vi "Save Best Fit Parameters.vi"(8 "Current File Num":i32, 9 "Best Fit Parameters":dbl[](array[numeric]), 10 "Fitting Results Save Path":string[](array[string]), 11 "Fitting Type":u16(ring)) -> ()   [LabVIEW 2013]
uses:
  <vilib>/Utility/file.llb/Read From Spreadsheet File (DBL).vi
  <vilib>/Utility/file.llb/Write To Spreadsheet File (DBL).vi
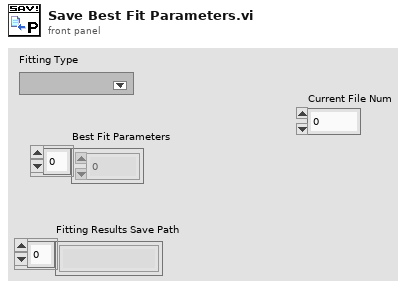
[diagram p1: front panel]
types:
  T1 = enum16{"open", "replace", "create", "open or create", "replace or create", "replace or create with confirmation"}
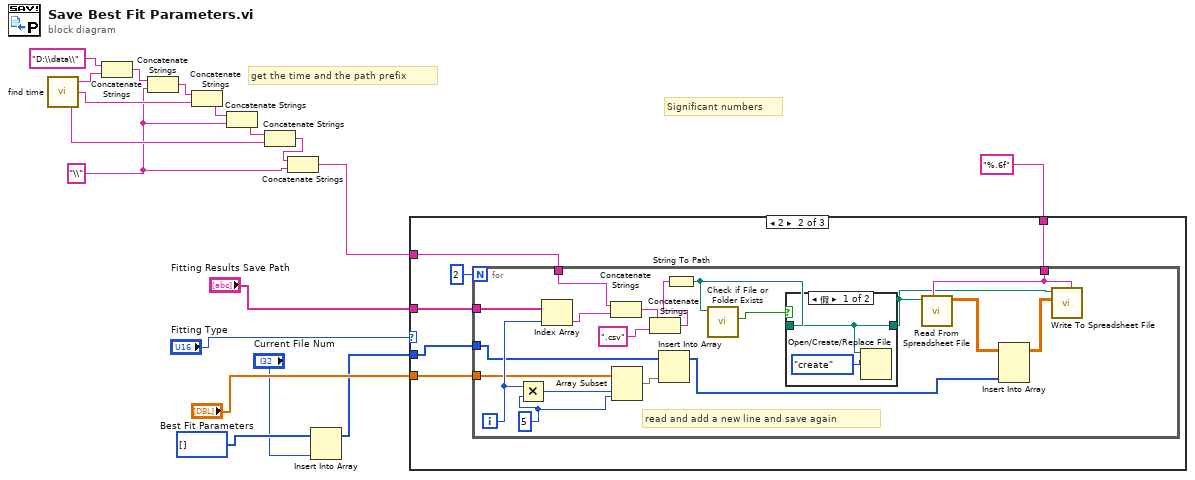
[diagram p0: block diagram]
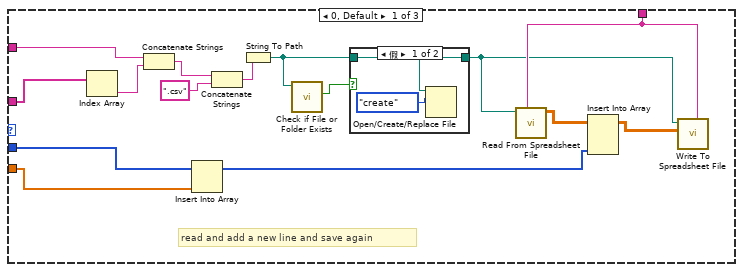
[diagram p2: hidden frame]
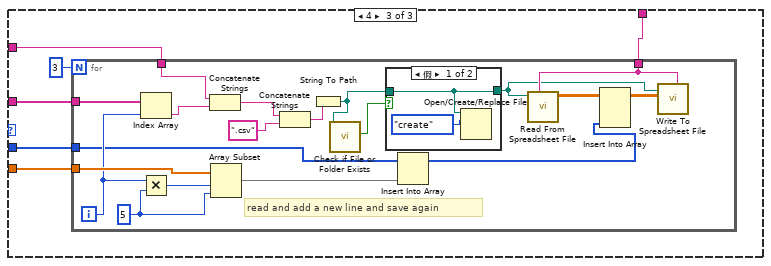
[diagram p5: hidden frame]
diagram:
  w2 = "\\" ("字符串")
  # "get the time and the path prefix"
  # "Significant numbers"
  n1 = call "find time.vi"() -> ("day"=w4:string, "month"=w7:string, "year"=w10:string)  [unwired: 3 in]
  n2 = Concatenate Strings("D:\\data\\", w10) -> (w9:string)
  n3 = Concatenate Strings(w9, w2) -> (w8:string)
  n4 = Concatenate Strings(w8, w7) -> (w6:string)
  n5 = Concatenate Strings(w6, w2) -> (w5:string)
  n6 = Concatenate Strings(w5, w4) -> (w3:string)
  n7 = Concatenate Strings(w3, w2) -> (w1:string)
  n8 = Insert Into Array(array=i32[] [], new element="Current File Num") -> (w13:i32[])  [unwired: 1 in]
  n9 = case shown="2" "Fitting Type" {
    tunnel: "Best Fit Parameters" -> [w28 w41 w69]
    tunnel: "Fitting Results Save Path" -> [w31 w40 w68]
    tunnel: w13 -> [w29 w39 w67]
    tunnel: "%.6f" ("format (%.3f)") -> [w26 w38 w66]
    tunnel: w1 -> [w25 w37 w65]
    frame 0, Default {
      # "read and add a new line and save again"
      n10 = Index Array(array=w31) -> (element=w30:string)  [unwired: 1 in]
      n11 = Concatenate Strings(w25, w30) -> (w23:string)
      n12 = Insert Into Array(array=w29, new element=w28) -> (w27:i32[])  [unwired: 1 in]
      n13 = Concatenate Strings(w23, ".csv" ("字符串")) -> (w22:string)
      n14 = String To Path(string=w22) -> (path=w21:path)
      n15 = call <vilib>:"Check if File or Folder Exists.vi"("path"=w21) -> ("file or folder exists?"=w19:bool)  [unwired: 8 in, 2 out]
      n16 = case shown="假" w19 {
        tunnel: w21 -> [w34 w36]
        tunnel: [w34 w36] -> w20
        frame False {
          n17 = Open/Create/Replace File(file path (use dialog)=w34, operation (0:open)=T1."create" ("操作(0:open)")) -> ()  [unwired: 4 in, 3 out]
        }
        frame True {
        }
      }
      n18 = call-poly <vilib>:"Read From Spreadsheet File.vi"("format (%.3f)"=w26, "file path (dialog if empty)"=w20) -> ("all rows"=w33:dbl[][])  [unwired: 5 in, 4 out]
      n19 = Insert Into Array(array=w33, new element=w27) -> (w32:dbl[][])  [unwired: 2 in]
      n20 = call-poly <vilib>:"Write To Spreadsheet File.vi"("format (%.3f)"=w26, "2D data"=w32, "file path (dialog if empty)"=w20) -> ()  [unwired: 5 in, 1 out]
    }
    frame 2 {
      n21 = for {
        N: 2 -> [_]
        tunnel: w41 -> [w53]
        tunnel: w40 -> [w59]
        tunnel: w39 -> [w54]
        tunnel: w38 -> [w50]
        tunnel: w37 -> [w49]
        i -> [w58]
        w60 = 5 ("x")
        # "read and add a new line and save again"
        n22 = Multiply(x=w58, y=w60) -> (x*y=w61:i32)
        n23 = Index Array(array=w59, index=w58) -> (element=w57:string)
        n24 = Concatenate Strings(w49, w57) -> (w48:string)
        n25 = Array Subset(array=w53, index=w61, length=w60) -> (w52:dbl[])
        n26 = Concatenate Strings(w48, ".csv" ("字符串")) -> (w46:string)
        n27 = Insert Into Array(array=w54, new element=w52) -> (w51:i32[])  [unwired: 1 in]
        n28 = String To Path(string=w46) -> (path=w45:path)
        n29 = call <vilib>:"Check if File or Folder Exists.vi"("path"=w45) -> ("file or folder exists?"=w43:bool)  [unwired: 8 in, 2 out]
        n30 = case shown="假" w43 {
          tunnel: w45 -> [w62 w64]
          tunnel: [w62 w64] -> w44
          frame False {
            n31 = Open/Create/Replace File(file path (use dialog)=w62, operation (0:open)=T1."create" ("操作(0:open)")) -> ()  [unwired: 4 in, 3 out]
          }
          frame True {
          }
        }
        n32 = call-poly <vilib>:"Read From Spreadsheet File.vi"("format (%.3f)"=w50, "file path (dialog if empty)"=w44) -> ("all rows"=w56:dbl[][])  [unwired: 5 in, 4 out]
        n33 = Insert Into Array(array=w56, new element=w51) -> (w55:dbl[][])  [unwired: 2 in]
        n34 = call-poly <vilib>:"Write To Spreadsheet File.vi"("format (%.3f)"=w50, "2D data"=w55, "file path (dialog if empty)"=w44) -> ()  [unwired: 5 in, 1 out]
      }
    }
    frame 4 {
      n35 = for {
        N: 3 -> [_]
        tunnel: w69 -> [w87]
        tunnel: w68 -> [w86]
        tunnel: w67 -> [w79]
        tunnel: w66 -> [w78]
        tunnel: w65 -> [w77]
        i -> [w85]
        w88 = 5 ("x")
        # "read and add a new line and save again"
        n36 = Index Array(array=w86, index=w85) -> (element=w84:string)
        n37 = Multiply(x=w85, y=w88) -> (x*y=w89:i32)
        n38 = Concatenate Strings(w77, w84) -> (w75:string)
        n39 = Array Subset(array=w87, index=w89, length=w88) -> (w81:dbl[])
        n40 = Concatenate Strings(w75, ".csv" ("字符串")) -> (w74:string)
        n41 = String To Path(string=w74) -> (path=w72:path)
        n42 = call <vilib>:"Check if File or Folder Exists.vi"("path"=w72) -> ("file or folder exists?"=w73:bool)  [unwired: 8 in, 2 out]
        n43 = case shown="假" w73 {
          tunnel: [w90 w92] -> w71
          tunnel: w72 -> [w90 w92]
          frame False {
            n44 = Open/Create/Replace File(file path (use dialog)=w90, operation (0:open)=T1."create" ("操作(0:open)")) -> ()  [unwired: 4 in, 3 out]
          }
          frame True {
          }
        }
        n45 = Insert Into Array(array=w79, new element=w81) -> (w80:i32[])  [unwired: 1 in]
        n46 = call-poly <vilib>:"Read From Spreadsheet File.vi"("format (%.3f)"=w78, "file path (dialog if empty)"=w71) -> ("all rows"=w83:dbl[][])  [unwired: 5 in, 4 out]
        n47 = Insert Into Array(array=w83, new element=w80) -> (w82:dbl[][])  [unwired: 2 in]
        n48 = call-poly <vilib>:"Write To Spreadsheet File.vi"("format (%.3f)"=w78, "2D data"=w82, "file path (dialog if empty)"=w71) -> ()  [unwired: 5 in, 1 out]
      }
    }
  }
